vi "Com_Base.vi"() -> ()   [LabVIEW 2019]
uses:
  MessageFormat1.ctl
  <vilib>/Instr/_visa.llb/VISA Configure Serial Port (Instr).vi
panel:
  in  "Disconnect from Arduino":bool
  out "Connected":bool
  in  "Connect to Arduino":bool
  in  "VISA resource name":refnum<visa-resource-name>
  out "Rx Number":u32
  in  "stop":bool
  out "Receiving Data":bool
  out "Input buffer":string
  in  "Stop Acquisition":bool
  in  "Start Acquisition":bool
  # "Dades rebudes per UART"
  # "Dades transportades al Consumer Loop"
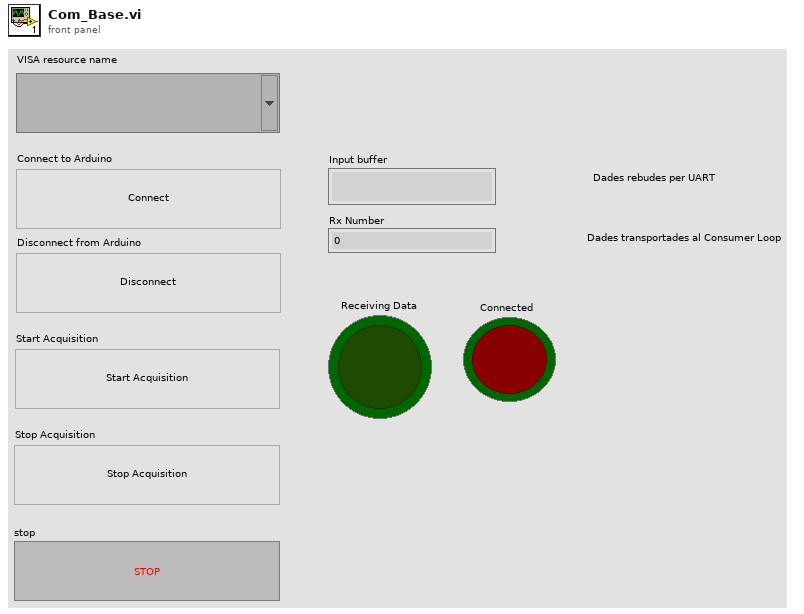
[diagram p1: front panel]
types:
  T1 = typedef "MessageFormat1.ctl" = cluster{"Consumer State":string, "RxData":string, "error constant":errorcluster, "Producer State ":string, "Numeric":dbl}
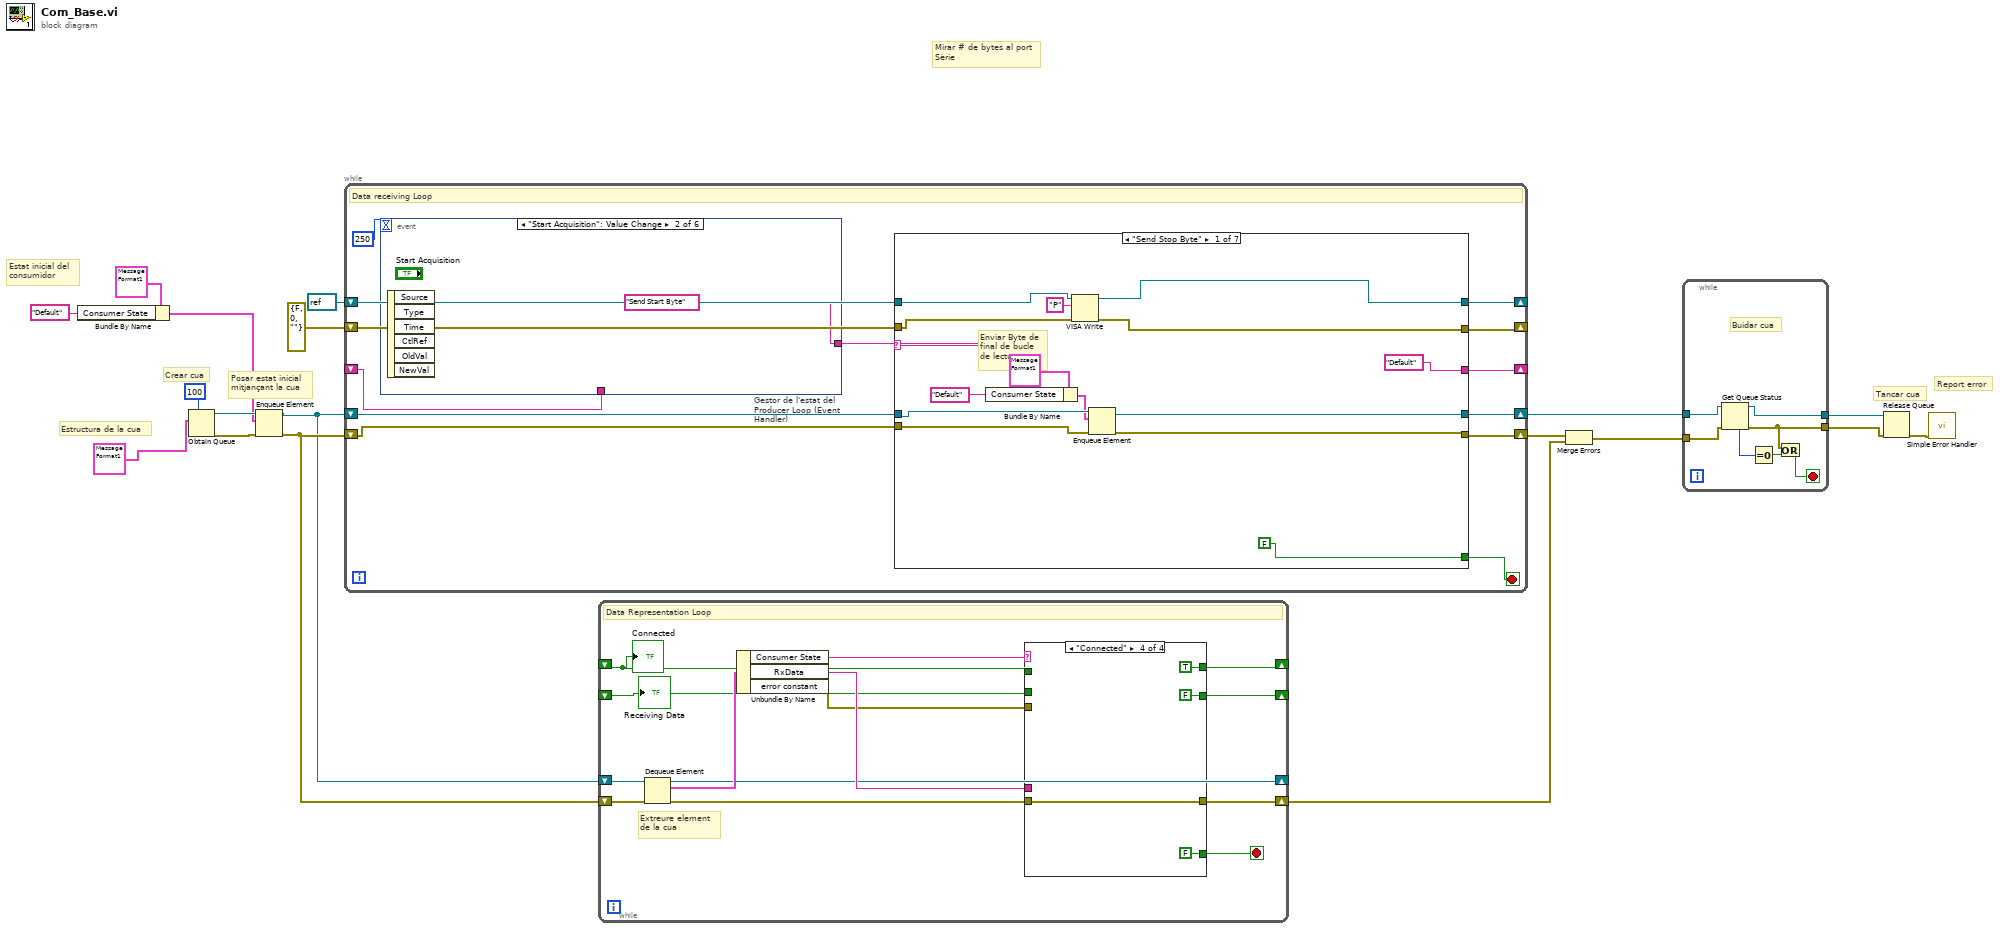
[diagram p0: block diagram]
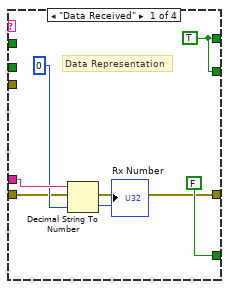
[diagram p2: hidden frame]
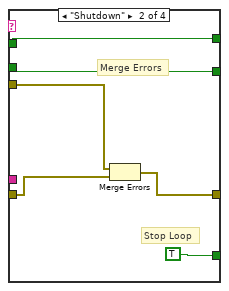
[diagram p3: hidden frame]
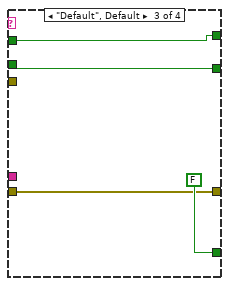
[diagram p4: hidden frame]
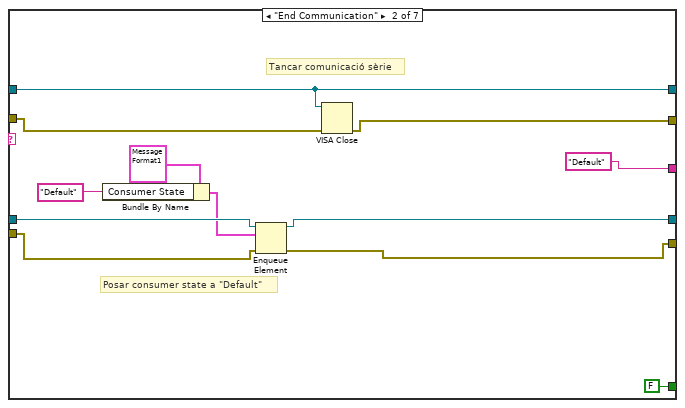
[diagram p5: hidden frame]
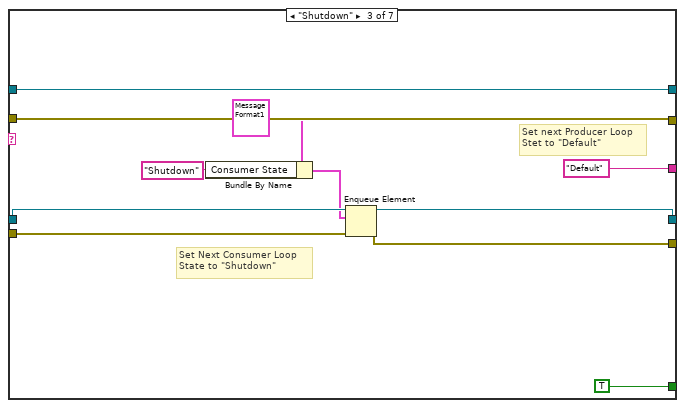
[diagram p6: hidden frame]
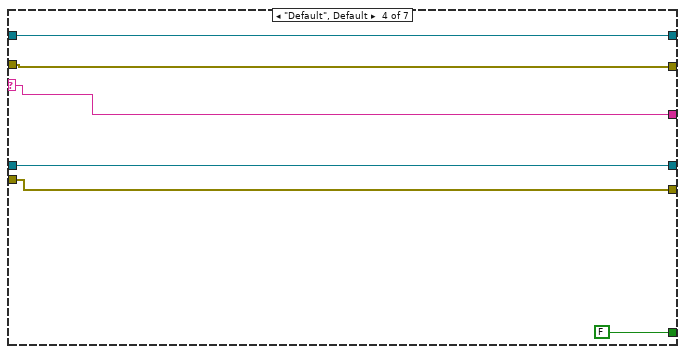
[diagram p7: hidden frame]
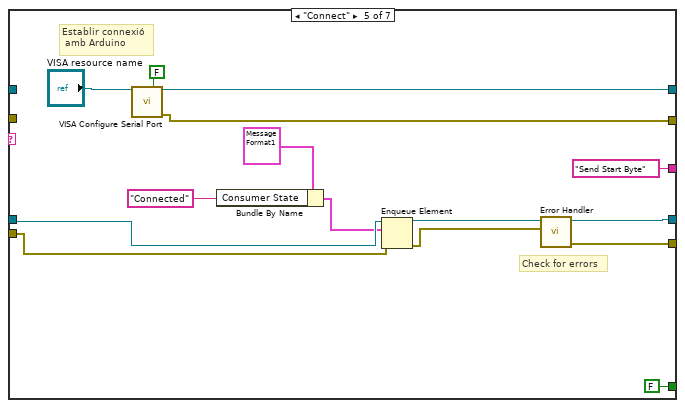
[diagram p8: hidden frame]
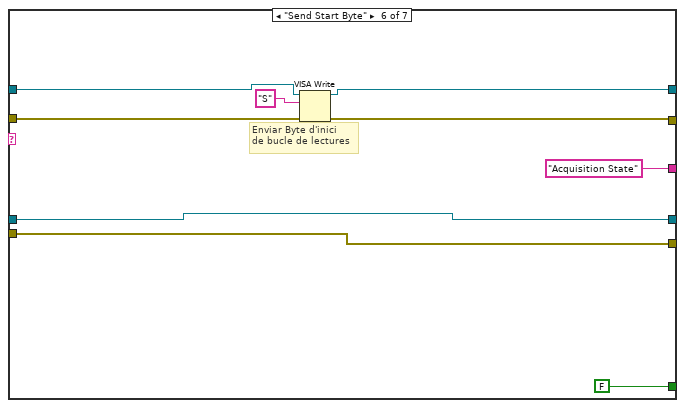
[diagram p9: hidden frame]
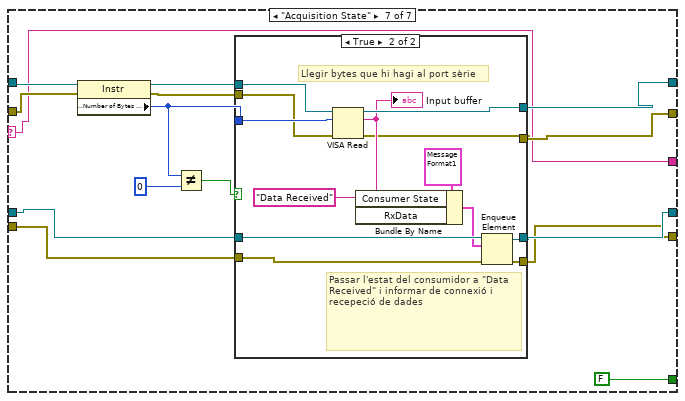
[diagram p10: hidden frame]
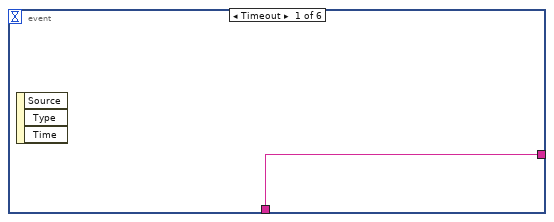
[diagram p12: hidden frame]
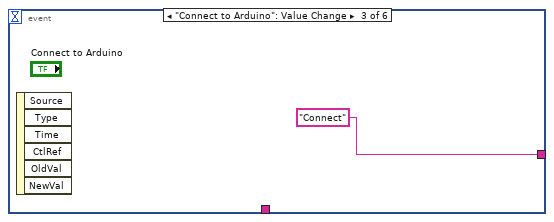
[diagram p13: hidden frame]
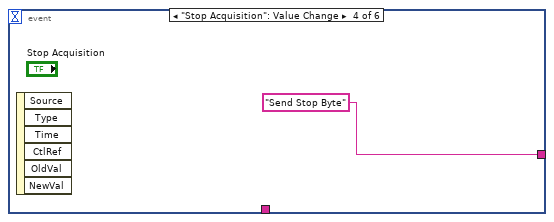
[diagram p14: hidden frame]
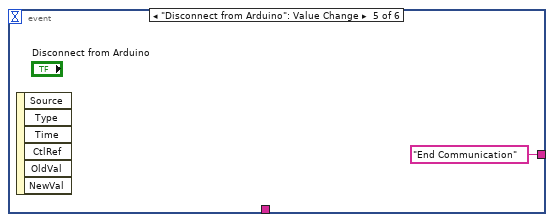
[diagram p15: hidden frame]
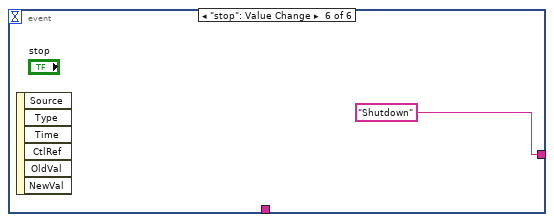
[diagram p16: hidden frame]
diagram:
  # "Tancar cua"
  # "Report error"
  # "Posar estat inicial \nmitjançant la cua"
  # "Crear cua"
  # "Mirar # de bytes al port\nSèrie"
  # "Estat inicial del \nconsumidor"
  # "Estructura de la cua"
  n1 = Bundle By Name(cluster=T1 {"Consumer State"="Consumer State", "RxData"="Received Data", "error constant"={"status"=FALSE, "code"=0, "source"=""}, "Producer State "="Consumer State", "Numeric"=0.0} ("Queue Definition"), "Consumer State"="Default") -> (w9:T1)
  n2 = Obtain Queue(max queue size (-1, unlimited)=100, element data type=T1 {"Consumer State"="Consumer State", "RxData"="Received Data", "error constant"={"status"=FALSE, "code"=0, "source"=""}, "Producer State "="Consumer State", "Numeric"=0.0} ("Queue Definition")) -> (queue out=w11:refnum<queue>, error out=w14:errorcluster)  [unwired: 3 in, 1 out]
  n3 = Enqueue Element(queue=w11, element=w9, error in (no error)=w14) -> (queue out=w12:refnum<queue>, error out=w13:errorcluster)  [unwired: 1 in, 1 out]
  n4 = while {
    shift-right: [w31] -> _
    shift-left: refnum<visa-resource-name> refnum ("VISA resource name out") -> [w26]
    shift-right: [w30] -> _
    shift-left: errorcluster {"status"=FALSE, "code"=0, "source"=""} ("error out") -> [w25]
    shift-right: [w19] -> w5
    shift-left: w12 -> [w22]
    shift-right: [w20] -> w17
    shift-left: w13 -> [w23]
    shift-right: [w27] -> _
    shift-left: _ -> [w24]
    stop <- w21 stop-if-true
    # "Data receiving Loop"
    n5 = event "Gestor de l'estat del Producer Loop (Event Handler)" shown="[1] \"Start Acquisition\": Value Change" {
      selector: _ -> [_ _ _ _ _ _]
      dyn-events: _ -> [_ _ _ _ _ _]
      timeout: 250 -> [_ _ _ _ _ _]
      tunnel: [w131 "Send Start Byte" "Connect" ("f") "Send Stop Byte" "End Communication" ("Producer State Out") "Shutdown"] -> w28
      tunnel: w24 -> [w131 _ _ _ _ _]
      event Timeout {
        n6 = event-data() -> ()  [unwired: 1 in, 3 out]
      }
      event "Start Acquisition": Value Change {
        n7 = event-data() -> ()  [unwired: 1 in, 6 out]
      }
      event "Connect to Arduino": Value Change {
        n8 = event-data() -> ()  [unwired: 1 in, 6 out]
      }
      event "Stop Acquisition": Value Change {
        n9 = event-data() -> ()  [unwired: 1 in, 6 out]
      }
      event "Disconnect from Arduino": Value Change {
        n10 = event-data() -> ()  [unwired: 1 in, 6 out]
      }
      event "stop": Value Change {
        n11 = event-data() -> ()  [unwired: 1 in, 6 out]
      }
    }
    n12 = case shown="\"Send Stop Byte\"" w28 {
      selector: w28 -> [_ _ _ w71 _ _ w101]
      tunnel: [w41 w55 w67 w72 w86 w95 w108] -> w31
      tunnel: [w40 w54 w66 w73 w83 w93 w102] -> w30
      tunnel: [w32 w48 w61 w74 w84 w92 w99] -> w20
      tunnel: [w33 w47 w62 w69 w85 w91 w100] -> w19
      tunnel: [FALSE FALSE TRUE FALSE FALSE FALSE FALSE] -> w21
      tunnel: ["Default" ("Producer State In") "Default" ("Producer State In") "Default" ("f") w71 "Send Start Byte" ("Producer State Out") "Acquisition State" ("Producer State In") w101] -> w27
      tunnel: w26 -> [w42 w55 w67 w72 _ w96 w113]
      tunnel: w25 -> [w43 w56 w66 w73 _ w97 w112]
      tunnel: w23 -> [w39 w52 w60 w74 w79 w92 w106]
      tunnel: w22 -> [w38 w53 w64 w69 w80 w91 w107]
      frame "Send Stop Byte" {
        # "Enviar Byte de \nfinal de bucle \nde lectures"
        n13 = Bundle By Name(cluster=T1 {"Consumer State"="Consumer State", "RxData"="Received Data", "error constant"={"status"=FALSE, "code"=0, "source"=""}, "Producer State "="Consumer State", "Numeric"=0.0} ("Queue Definition"), "Consumer State"="Default") -> (w37:T1)
        n14 = VISA Write(VISA resource name=w42, write buffer="P", error in (no error)=w43) -> (VISA resource name out=w41:refnum<visa-resource-name>, error out=w40:errorcluster)  [unwired: 1 out]
        n15 = Enqueue Element(queue=w38, element=w37, error in (no error)=w39) -> (queue out=w33:refnum<queue>, error out=w32:errorcluster)  [unwired: 1 in, 1 out]
      }
      frame "End Communication" {
        # "Tancar comunicació sèrie"
        # "Posar consumer state a \"Default\""
        n16 = Bundle By Name(cluster=T1 {"Consumer State"="Consumer State", "RxData"="Received Data", "error constant"={"status"=FALSE, "code"=0, "source"=""}, "Producer State "="Consumer State", "Numeric"=0.0} ("Queue Definition"), "Consumer State"="Default") -> (w49:T1)
        n17 = Enqueue Element(queue=w53, element=w49, error in (no error)=w52) -> (queue out=w47:refnum<queue>, error out=w48:errorcluster)  [unwired: 1 in, 1 out]
        n18 = VISA Close(VISA resource name=w55, error in (no error)=w56) -> (error out=w54:errorcluster)
      }
      frame "Shutdown" {
        # "Set next Producer Loop\nStet to \"Default\""
        # "Set Next Consumer Loop\nState to \"Shutdown\""
        n19 = Bundle By Name(cluster=T1 {"Consumer State"="Consumer State", "RxData"="Received Data", "error constant"={"status"=FALSE, "code"=0, "source"=""}, "Producer State "="Consumer State", "Numeric"=0.0} ("Queue Definition"), "Consumer State"="Shutdown") -> (w58:T1)
        n20 = Enqueue Element(queue=w64, element=w58, error in (no error)=w60) -> (queue out=w62:refnum<queue>, error out=w61:errorcluster)  [unwired: 1 in, 1 out]
      }
      frame "Default", Default {
      }
      frame "Connect" {
        # "Check for errors"
        # "Establir connexió\n amb Arduino"
        n21 = call-poly "VISA Configure Serial Port"("VISA resource name"="VISA resource name", "Enable Termination\nChar (T)"=FALSE ("Enable Termination\nChar (T)")) -> ("VISA resource name out"=w86:refnum<visa-resource-name>, "error out"=w83:errorcluster)  [unwired: 12 in]
        n22 = Bundle By Name(cluster=T1 {"Consumer State"="Consumer State", "RxData"="Received Data", "error constant"={"status"=FALSE, "code"=0, "source"=""}, "Producer State "="Consumer State", "Numeric"=0.0} ("Queue Definition"), "Consumer State"="Connected") -> (w76:T1)
        n23 = Enqueue Element(queue=w80, element=w76, error in (no error)=w79) -> (queue out=w81:refnum<queue>, error out=w82:errorcluster)  [unwired: 1 in, 1 out]
        n24 = call "Error Handler.vi"("error in"=w82, "Queue in"=w81) -> ("error out"=w84:errorcluster, "Queue out"=w85:refnum<queue>)  [unwired: 8 in]
      }
      frame "Send Start Byte" {
        # "Enviar Byte d'inici\nde bucle de lectures"
        n25 = VISA Write(VISA resource name=w96, write buffer="S", error in (no error)=w97) -> (VISA resource name out=w95:refnum<visa-resource-name>, error out=w93:errorcluster)  [unwired: 1 out]
      }
      frame "Acquisition State" {
        n26 = property class="Instr"(reference=w113, error in=w112) -> (reference out=w105:refnum<visa-resource-name>, error out=w104:errorcluster, "Serial Settings:Number of Bytes at Serial Port"=w111:u32)
        n27 = Not Equal?(x=w111, y=u32 0) -> (x != y?=w109:bool)
        n28 = case shown="True" w109 {
          tunnel: [w116 w130] -> w108
          tunnel: [w115 w120] -> w102
          tunnel: [w117 w119] -> w100
          tunnel: w111 -> [_ w127]
          tunnel: w107 -> [w117 w123]
          tunnel: w106 -> [w114 w124]
          tunnel: w105 -> [w116 w126]
          tunnel: w104 -> [w115 w125]
          tunnel: [w114 w118] -> w99
          frame False {
          }
          frame True {
            # "Passar l'estat del consumidor a \"Data Received\" i informar de connexió i recepeció de dades"
            # "Llegir bytes que hi hagi al port sèrie"
            n29 = VISA Read(VISA resource name=w126, byte count=w127, error in (no error)=w125) -> (VISA resource name out=w130:refnum<visa-resource-name>, read buffer=w129:string, error out=w120:errorcluster)  [unwired: 1 out]
            "Input buffer" <- w129
            n30 = Bundle By Name(cluster=T1 {"Consumer State"="Consumer State", "RxData"="Received Data", "error constant"={"status"=FALSE, "code"=0, "source"=""}, "Producer State "="Consumer State", "Numeric"=0.0} ("Queue Definition"), "Consumer State"="Data Received" ("Next State"), "RxData"=w129) -> (w121:T1)
            n31 = Enqueue Element(queue=w123, element=w121, error in (no error)=w124) -> (queue out=w119:refnum<queue>, error out=w118:errorcluster)  [unwired: 1 in, 1 out]
          }
        }
      }
    }
  }
  n32 = while {
    shift-right: [w142] -> w15
    shift-left: w13 -> [w149]
    shift-right: [w145] -> _
    shift-left: w12 -> [w150]
    shift-right: [w140] -> _
    shift-left: _ -> [w138]
    shift-right: [w139] -> _
    shift-left: _ -> [w137]
    stop <- w144 stop-if-true
    # "Extreure element \nde la cua"
    # "Data Representation Loop"
    n33 = Dequeue Element(queue=w150, error in (no error)=w149) -> (queue out=w145:refnum<queue>, element=w148:T1, error out=w141:errorcluster)  [unwired: 1 in, 1 out]
    n34 = Unbundle By Name(w148) -> ("Consumer State"=w146:string, "RxData"=w147:string, "error constant"=w143:errorcluster)
    n35 = case shown="\"Connected\"" w146 {
      tunnel: w147 -> [w155 _ _ _]
      tunnel: [FALSE TRUE FALSE FALSE] -> w144
      tunnel: w143 -> [_ w160 _ _]
      tunnel: [w152 w161 w165 w168] -> w142
      tunnel: w141 -> [w152 w159 w165 w168]
      tunnel: [w151 w158 w163 TRUE] -> w140
      tunnel: [w151 w157 w164 FALSE] -> w139
      tunnel: w138 -> [_ w158 w163 _]
      tunnel: w137 -> [_ w157 w164 _]
      frame "Data Received" {
        w151 = TRUE
        # "Data Representation"
        n36 = Decimal String To Number(string=w155, default (0L)=u32 0) -> (number=→"Rx Number":u32)  [unwired: 1 in, 1 out]
      }
      frame "Shutdown" {
        # "Stop Loop"
        # "Merge Errors"
        n37 = Merge Errors(w160, w159) -> (w161:errorcluster)
      }
      frame "Default", Default {
      }
      frame "Connected" {
      }
    }
    "Receiving Data" <- w137
    "Connected" <- w138
  }
  n38 = Merge Errors(w17, w15) -> (w4:errorcluster)
  n39 = while {
    tunnel: w5 -> [w177]
    tunnel: w4 -> [w176]
    tunnel: [w172] -> w3
    tunnel: [w175] -> w2
    stop <- w171 stop-if-true
    # "Buidar cua"
    n40 = Get Queue Status(queue=w177, error in (no error)=w176) -> (queue out=w175:refnum<queue>, error out=w172:errorcluster, # elements in queue=w174:i32)  [unwired: 1 in, 5 out]
    n41 = Equal To 0?(x=w174) -> (x = 0?=w173:bool)
    n42 = Or(x=w172, y=w173) -> (x .or. y?=w171:bool)
  }
  n43 = Release Queue(queue=w2, error in (no error)=w3) -> (error out=w1:errorcluster)  [unwired: 1 in, 2 out]
  n44 = call <vilib>:"Simple Error Handler.vi"("error in (no error)"=w1) -> ()  [unwired: 4 in, 5 out]
